vi "CRYAPI MANAGER LIB.vi"(4 "sOption":string, 8 "tFrame":T2, 9 "sData":string, 10 "nData":i32, 11 "sAction":string) -> (1 "nData_Out":i32, 2 "sData_Out":string, 3 "tFrame_Out":T2)   [LabVIEW 2013]
uses:
  <vilib>/Utility/miscctls.llb/LVRectTypeDef.ctl
  CRYMain Sub Window Global.vi
  CRYStepSetup/CRYStepSetup Global.vi
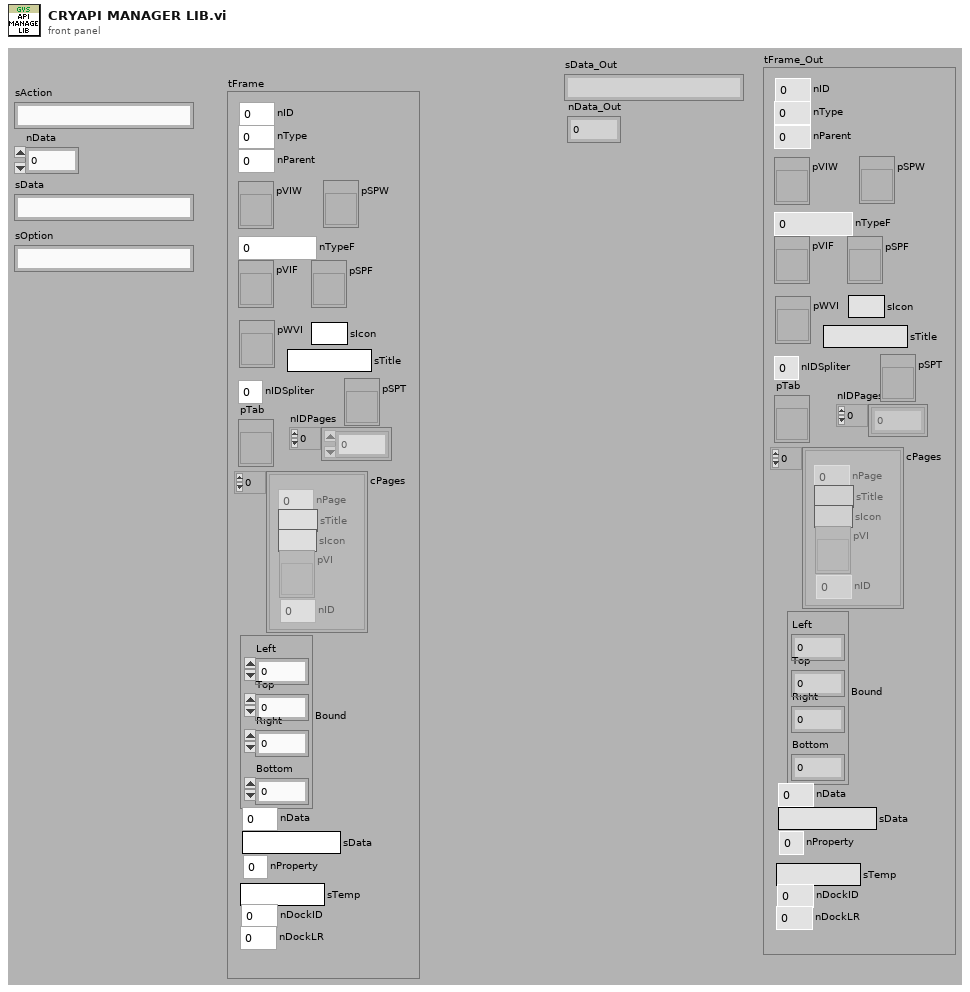
[diagram p1: front panel]
types:
  T1 = typedef "LVRectTypeDef.ctl" = cluster{"Left":i16, "Top":i16, "Right":i16, "Bottom":i16}
  T2 = cluster{"nType":i32, "nParent":i32, "pVIW":refnum<vi>, "pSPW":refnum<vi>, "nTypeF":i32, "pVIF":refnum<vi>, "pSPF":refnum<vi>, "nIDSpliter":i32, "nProperty":i32, "Bound":T1, "nID":i32, "nData":i32, "sData":string, "pWVI":refnum<vi>, "sTitle":string, "cPages":cluster{"nPage":i32, "sTitle":string, "sIcon":string, "pVI":refnum<vi>, "nID":i32}[], "pTab":refnum<vi>, "nIDPages":i32[], "pSPT":refnum<vi>, "sTemp":string, "nDockID":i32, "nDockLR":i32, "sIcon":string}
  T3 = cluster{"nID":i32[], "Frame":cluster{"nType":i32, "nParent":i32, "pVIW":refnum<vi>, "pSPW":refnum<vi>, "nTypeF":i32, "pVIF":refnum<vi>, "pSPF":refnum<vi>, "nIDSpliter":i32, "nProperty":i32, "Bound":T1, "nID":i32, "nData":i32, "sData":string, "pWVI":refnum<vi>, "sTitle":string, "cPages":cluster{"nPage":i32, "sTitle":string, "sIcon":string, "pVI":refnum<vi>, "nID":i32}[], "pTab":refnum<vi>, "nIDPages":i32[], "pSPT":refnum<vi>, "sTemp":string, "nDockID":i32, "nDockLR":i32, "sIcon":string}[]}
  T4 = cluster{"nPos":i32, "Rect":T1, "Sizing":enum16{"Sticks Top/Left", "Sticks Bottom/Right", "Proportional"}}[]
  T5 = cluster{"nPos":i32, "Rect":T1, "Sizing":enum16{"Sticks Top/Left", "Sticks Bottom/Right", "Proportional"}}
  T6 = enum16{"Sticks Top/Left", "Sticks Bottom/Right", "Proportional"}
  T7 = enum32{"Invalid", "Standard", "Closed", "Hidden", "Minimized", "Maximized"}
  T8 = cluster{"nID":i32[], "Spliter":cluster{"nType":i32, "nTypeP":i32, "pVI":refnum<vi>, "pSpliter":refnum<vi>, "pSPL":refnum<vi>, "pVIL":refnum<vi>, "pSPR":refnum<vi>, "pVIR":refnum<vi>, "nIDTL":i32, "nIDL":i32, "nIDTR":i32, "nIDR":i32, "nID":i32, "nIDParent":i32, "nData":i32, "sData":string}[]}
  T9 = cluster{"nType":i32, "nTypeP":i32, "pVI":refnum<vi>, "pSpliter":refnum<vi>, "pSPL":refnum<vi>, "pVIL":refnum<vi>, "pSPR":refnum<vi>, "pVIR":refnum<vi>, "nIDTL":i32, "nIDL":i32, "nIDTR":i32, "nIDR":i32, "nID":i32, "nIDParent":i32, "nData":i32, "sData":string}[]
  T10 = cluster{"nType":i32, "nParent":i32, "pVIW":refnum<vi>, "pSPW":refnum<vi>, "nTypeF":i32, "pVIF":refnum<vi>, "pSPF":refnum<vi>, "nIDSpliter":i32, "nProperty":i32, "Bound":T1, "nID":i32, "nData":i32, "sData":string, "pWVI":refnum<vi>, "sTitle":string, "cPages":cluster{"nPage":i32, "sTitle":string, "sIcon":string, "pVI":refnum<vi>, "nID":i32}[], "pTab":refnum<vi>, "nIDPages":i32[], "pSPT":refnum<vi>, "sTemp":string, "nDockID":i32, "nDockLR":i32, "sIcon":string}[]
  T11 = typedef "CRYWindows Sysem.ctl" = cluster{"cFrame":cluster{"nID":i32[], "Frame":cluster{"nType":i32, "nParent":i32, "pVIW":refnum<vi>, "pSPW":refnum<vi>, "nTypeF":i32, "pVIF":refnum<vi>, "pSPF":refnum<vi>, "nIDSpliter":i32, "nProperty":i32, "Bound":T1, "nID":i32, "nData":i32, "sData":string, "pWVI":refnum<vi>, "sTitle":string, "cPages":cluster{"nPage":i32, "sTitle":string, "sIcon":string, "pVI":refnum<vi>, "nID":i32}[], "pTab":refnum<vi>, "nIDPages":i32[], "pSPT":refnum<vi>, "sTemp":string, "nDockID":i32, "nDockLR":i32, "sIcon":string}[]}, "cSpliter":cluster{"nID":i32[], "Spliter":cluster{"nType":i32, "nTypeP":i32, "pVI":refnum<vi>, "pSpliter":refnum<vi>, "pSPL":refnum<vi>, "pVIL":refnum<vi>, "pSPR":refnum<vi>, "pVIR":refnum<vi>, "nIDTL":i32, "nIDL":i32, "nIDTR":i32, "nIDR":i32, "nID":i32, "nIDParent":i32, "nData":i32, "sData":string}[]}, "ActiveWID":i32, "cSpliterPos":cluster{"nPos":i32, "Rect":T1, "Sizing":enum16{"Sticks Top/Left", "Sticks Bottom/Right", "Proportional"}}[], "CounterWID":i32, "CounterActive":i32, "CounterSpliter":i32, "cWinStatus":cluster{"nData":i32, "nActiveNum":i32}[], "StepName":string, "StepVINo":i32}
  T12 = cluster{"sStepName":string, "nStepVINo":i32, "nStepVINoDisplay":i32}
  T13 = cluster{"nType":i32, "nTypeP":i32, "pVI":refnum<vi>, "pSpliter":refnum<vi>, "pSPL":refnum<vi>, "pVIL":refnum<vi>, "pSPR":refnum<vi>, "pVIR":refnum<vi>, "nIDTL":i32, "nIDL":i32, "nIDTR":i32, "nIDR":i32, "nID":i32, "nIDParent":i32, "nData":i32, "sData":string}
  T14 = cluster{"CLOSE_HIDE":i32, "CLOSE_CLOSE":i32, "DOCK_ENABLE":i32, "DOCK_DISABLE":i32, "FOCUS_SHOW":i32, "FOCUS_HIDE":i32}
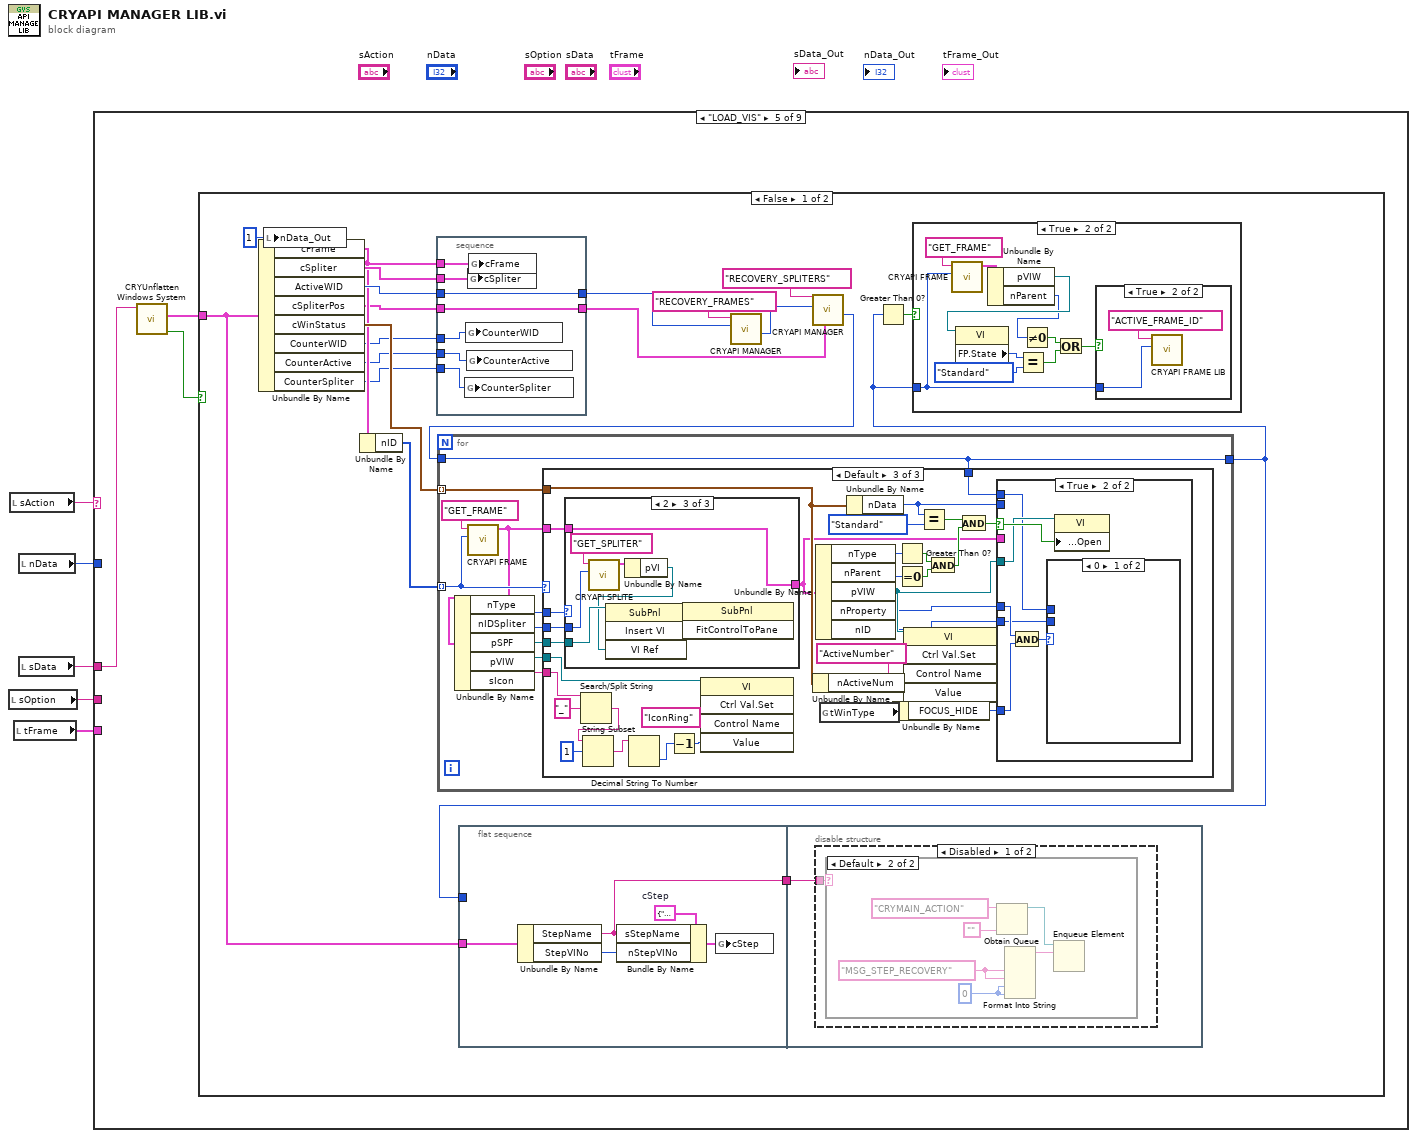
[diagram p0: block diagram]
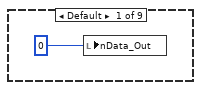
[diagram p2: hidden frame]
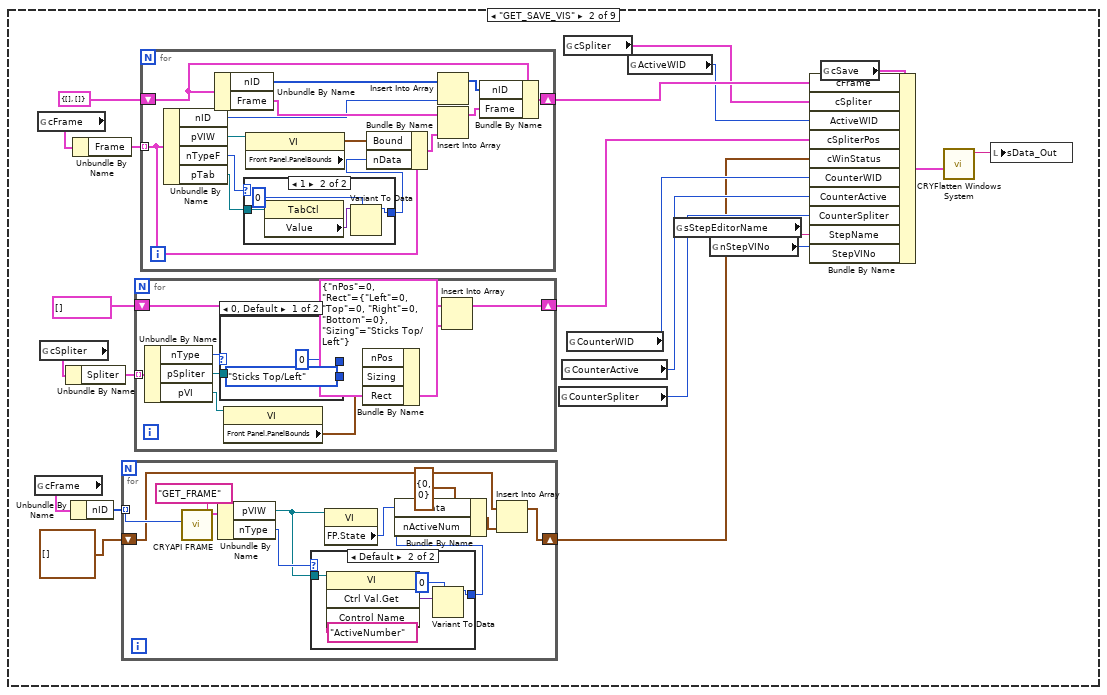
[diagram p3: hidden frame]
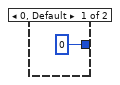
[diagram p4: hidden frame]
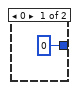
[diagram p5: hidden frame]
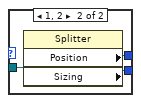
[diagram p6: hidden frame]
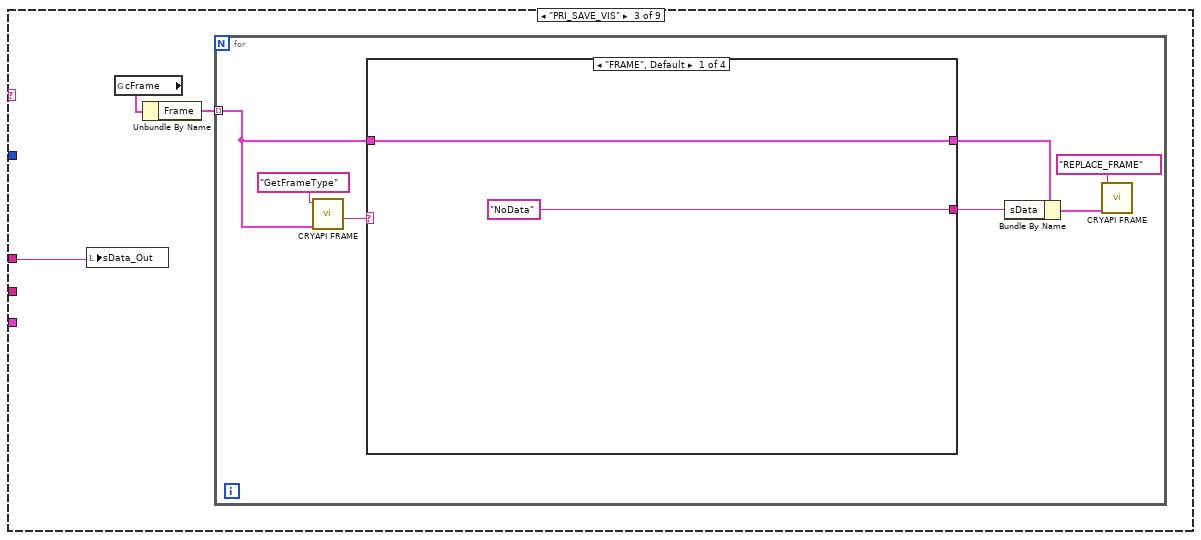
[diagram p7: hidden frame]
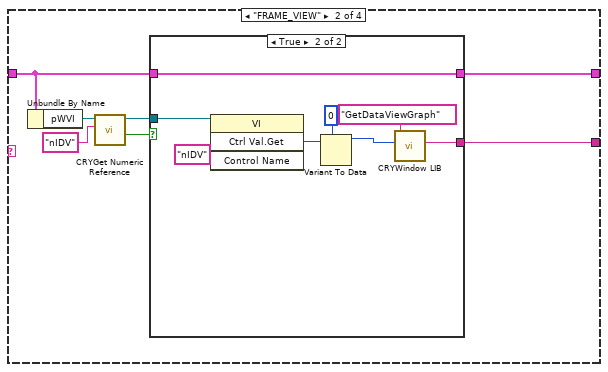
[diagram p8: hidden frame]
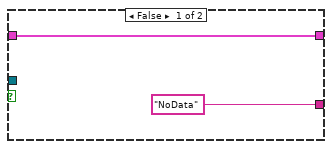
[diagram p9: hidden frame]
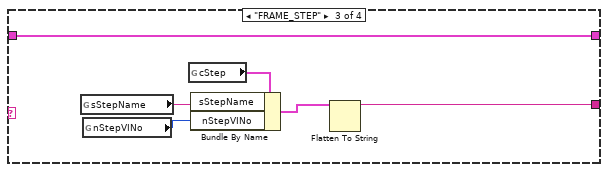
[diagram p10: hidden frame]
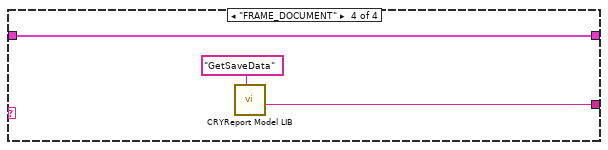
[diagram p11: hidden frame]
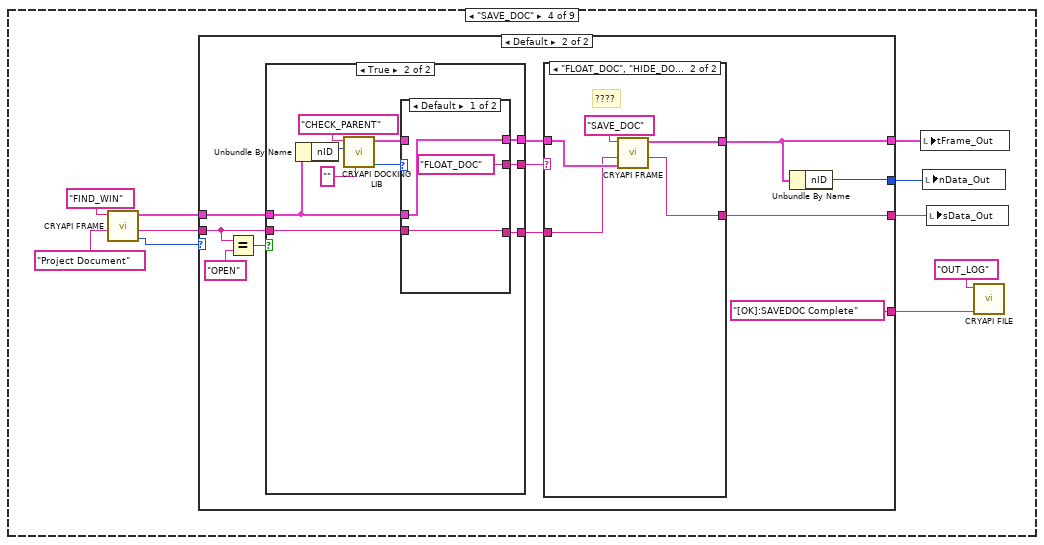
[diagram p12: hidden frame]
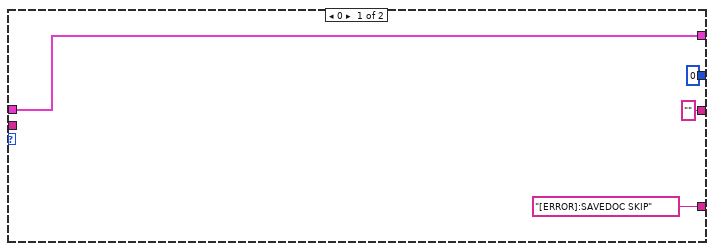
[diagram p13: hidden frame]
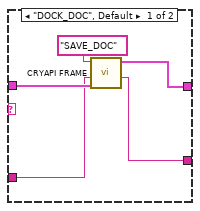
[diagram p14: hidden frame]
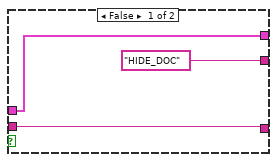
[diagram p15: hidden frame]
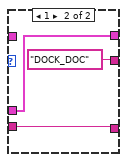
[diagram p16: hidden frame]
diagram:
  n1 = local read "sOption"() -> (w1:string)
  n2 = local read "sAction"() -> (w5:string)
  n3 = local read "tFrame"() -> (w3:T2)
  n4 = local read "nData"() -> (w4:i32)
  n5 = local read "sData"() -> (w2:string)
  n6 = case shown="\"LOAD_VIS\"" w5 {
    selector: w5 -> [_ _ _ _ _ w324 _ _ _]
    tunnel: w4 -> [_ _ _ _ _ _ _ _ _]
    tunnel: w2 -> [_ _ w81 _ w175 w323 _ _ w350]
    tunnel: w3 -> [_ _ _ _ _ w322 _ _ _]
    tunnel: w1 -> [_ _ _ _ _ _ _ _ w348]
    frame Default {
      n7 = local write "nData_Out"(0 ("nData_Out")) -> ()
    }
    frame "GET_SAVE_VIS" {
      n8 = global read "CRYMain Sub Window Global.vi" "cFrame"() -> (w18:T3)
      n9 = global read "CRYMain Sub Window Global.vi" "cFrame"() -> (w22:T3)
      n10 = global read "CRYMain Sub Window Global.vi" "cSpliter"() -> (w14:T8)
      n11 = Unbundle By Name(w14) -> ("Spliter"=w15:T9)
      n12 = Unbundle By Name(w18) -> ("nID"=w17:i32[])
      n13 = Unbundle By Name(w22) -> ("Frame"=w21:T10)
      n14 = for {
        shift-right: [w54] -> w19
        shift-left: cluster{"nData":i32, "nActiveNum":i32}[] [] ("cWinStatus") -> [w55]
        tunnel: w17 -> [w57] mode=indexing
        n15 = call "CRYAPI FRAME.vi"("nData"=w57, "sAction"="GET_FRAME") -> ("tFrame_Out"=w56:T2)  [unwired: 4 in, 5 out]
        n16 = Unbundle By Name(w56) -> ("pVIW"=w48:refnum<vi>, "nType"=w51:i32)
        n17 = case shown="Default" w51 {
          tunnel: [0 ("Numeric") w61] -> w50
          tunnel: w48 -> [_ w60]
          frame 0 {
          }
          frame Default {
            n18 = invoke class="VI" method="Ctrl Val.Get"(reference=w60, "Control Name"="ActiveNumber") -> ("Get Control Value Variant"=w62:variant)  [unwired: 2 in, 3 out]
            n19 = Variant To Data(type=0 ("Numeric"), Variant=w62) -> (data=w61:i32)  [unwired: 1 in, 1 out]
          }
        }
        n20 = property class="VI"(reference=w48) -> ("FP.State"=w49:T7)  [unwired: 1 in, 2 out]
        n21 = Bundle By Name(cluster=cluster{"nData":i32, "nActiveNum":i32} {"nData"=0, "nActiveNum"=0} ("tWinStatus"), "nData"=w49, "nActiveNum"=w50) -> (w52:cluster{"nData":i32, "nActiveNum":i32})
        n22 = Insert Into Array(array=w55, new element=w52) -> (w54:cluster{"nData":i32, "nActiveNum":i32}[])  [unwired: 1 in]
      }
      n23 = for {
        shift-right: [w73] -> w16
        shift-left: T4 [] ("nSpliterPos") -> [w74]
        tunnel: w15 -> [w71] mode=indexing
        n24 = Unbundle By Name(w71) -> ("nType"=w75:i32, "pSpliter"=w72:refnum<vi>, "pVI"=w70:refnum<vi>)
        n25 = case shown="0, Default" w75 {
          tunnel: w72 -> [_ w80]
          tunnel: [0 ("Position") w79] -> w69
          tunnel: [T6."Sticks Top/Left" ("Sizing") w78] -> w65
          frame 0, Default {
          }
          frame 1, 2 {
            n26 = property class="Splitter"(reference=w80) -> ("Position"=w79:i32, "Sizing"=w78:T6)  [unwired: 1 in, 2 out]
          }
        }
        n27 = property class="VI"(reference=w70) -> ("Front Panel.PanelBounds"=w68:T1)  [unwired: 1 in, 2 out]
        n28 = Bundle By Name(cluster=T5 {"nPos"=0, "Rect"={"Left"=0, "Top"=0, "Right"=0, "Bottom"=0}, "Sizing"=enum."Sticks Top/Left"} ("tSpliterSave"), "nPos"=w69, "Sizing"=w65, "Rect"=w68) -> (w67:T5)
        n29 = Insert Into Array(array=w74, new element=w67) -> (w73:T4)  [unwired: 1 in]
      }
      n30 = for {
        tunnel: w21 -> [w41] mode=indexing
        shift-right: [w32] -> w23
        shift-left: T3 {"nID"=[], "Frame"=[]} ("cFrame") -> [w35]
        n31 = Unbundle By Name(w41) -> ("nID"=w36:i32, "pVIW"=w42:refnum<vi>, "nTypeF"=w31:i32, "pTab"=w30:refnum<vi>)
        n32 = Unbundle By Name(w35) -> ("nID"=w39:i32[], "Frame"=w38:T10)
        n33 = case shown="1" w31 {
          tunnel: [0 w46] -> w29
          tunnel: w30 -> [_ w45]
          frame 0, Default {
          }
          frame 1 {
            n34 = property class="TabCtl"(reference=w45) -> ("Value"=w44:variant)  [unwired: 1 in, 2 out]
            n35 = Variant To Data(type=0, Variant=w44) -> (data=w46:i32)  [unwired: 1 in, 1 out]
          }
        }
        n36 = property class="VI"(reference=w42) -> ("Front Panel.PanelBounds"=w40:T1)  [unwired: 1 in, 2 out]
        n37 = Bundle By Name(cluster=w41, "Bound"=w40, "nData"=w29) -> (w37:T2)
        n38 = Insert Into Array(array=w39, new element=w36) -> (w34:i32[])  [unwired: 1 in]
        n39 = Insert Into Array(array=w38, new element=w37) -> (w33:T10)  [unwired: 1 in]
        n40 = Bundle By Name(cluster=w35, "nID"=w34, "Frame"=w33) -> (w32:T3)
      }
      n41 = global read "CRYMain Sub Window Global.vi" "CounterSpliter"() -> (w26:i32)
      n42 = global read "CRYMain Sub Window Global.vi" "CounterActive"() -> (w25:i32)
      n43 = global read "CRYMain Sub Window Global.vi" "cSpliter"() -> (w12:T8)
      n44 = global read "CRYMain Sub Window Global.vi" "CounterWID"() -> (w24:i32)
      n45 = global read "CRYMain Sub Window Global.vi" "ActiveWID"() -> (w13:i32)
      n46 = global read "CRYStepSetup Global.vi" "sStepEditorName"() -> (w8:string)
      n47 = global read "CRYStepSetup Global.vi" "nStepVINo"() -> (w7:i32)
      n48 = global read "CRYMain Sub Window Global.vi" "cSave"() -> (w11:T11)
      n49 = Bundle By Name(cluster=w11, "cFrame"=w23, "cSpliter"=w12, "ActiveWID"=w13, "cSpliterPos"=w16, "cWinStatus"=w19, "CounterWID"=w24, "CounterActive"=w25, "CounterSpliter"=w26, "StepName"=w8, "StepVINo"=w7) -> (w10:T11)
      n50 = call "CRYFlatten Windows System.vi"("Windows System"=w10) -> ("WinSys flattened"=w9:string)  [unwired: 10 in]
      n51 = local write "sData_Out"(w9) -> ()
    }
    frame "PRI_SAVE_VIS" {
      n52 = local write "sData_Out"(w81) -> ()
      n53 = global read "CRYMain Sub Window Global.vi" "cFrame"() -> (w83:T3)
      n54 = Unbundle By Name(w83) -> ("Frame"=w82:T10)
      n55 = for {
        tunnel: w82 -> [w89] mode=indexing
        n56 = call "CRYAPI FRAME.vi"("tFrame"=w89, "sAction"="GetFrameType") -> ("sData_Out"=w88:string)  [unwired: 6 in, 3 out]
        n57 = case shown="\"FRAME\", Default" w88 {
          tunnel: w89 -> [w92 w95 w115 w118]
          tunnel: [w92 w94 w115 w118] -> w84
          tunnel: ["NoData" ("sData_Out") w93 w110 w116] -> w87
          frame "FRAME", Default {
          }
          frame "FRAME_VIEW" {
            n58 = Unbundle By Name(w95) -> ("pWVI"=w98:refnum<vi>)
            n59 = call "CRYGet Numeric Reference.vi"("Label Name"="nIDV", "VI Refnum"=w98) -> ("Boolean"=w97:bool, "VI Refnum Out"=w96:refnum<vi>)  [unwired: 7 in, 1 out]
            n60 = case shown="True" w97 {
              tunnel: w96 -> [_ w107]
              tunnel: w95 -> [w101 w104]
              tunnel: ["NoData" ("sData_Out") w105] -> w93
              tunnel: [w101 w104] -> w94
              frame False {
              }
              frame True {
                n61 = invoke class="VI" method="Ctrl Val.Get"(reference=w107, "Control Name"="nIDV") -> ("Get Control Value Variant"=w109:variant)  [unwired: 2 in, 3 out]
                n62 = Variant To Data(type=0, Variant=w109) -> (data=w102:i32)  [unwired: 1 in, 1 out]
                n63 = call "CRYWindow LIB.vi"("nData"=w102, "sAction"="GetDataViewGraph") -> ("sData_Out"=w105:string)  [unwired: 9 in]
              }
            }
          }
          frame "FRAME_STEP" {
            n64 = global read "CRYStepSetup Global.vi" "sStepName"() -> (w113:string)
            n65 = global read "CRYStepSetup Global.vi" "nStepVINo"() -> (w112:i32)
            n66 = global read "CRYStepSetup Global.vi" "cStep"() -> (w114:T12)
            n67 = Bundle By Name(cluster=w114, "sStepName"=w113, "nStepVINo"=w112) -> (w111:T12)
            n68 = Flatten To String(anything=w111) -> (data string=w110:string)  [unwired: 1 in, 4 out]
          }
          frame "FRAME_DOCUMENT" {
            n69 = call "CRYReport Model LIB.vi"("sAction"="GetSaveData") -> ("sData_Out"=w116:string)  [unwired: 9 in, 1 out]
          }
        }
        n70 = Bundle By Name(cluster=w84, "sData"=w87) -> (w85:T2)
        n71 = call "CRYAPI FRAME.vi"("tFrame"=w85, "sAction"="REPLACE_FRAME") -> ()  [unwired: 6 in, 4 out]
      }
    }
    frame "SAVE_DOC" {
      n72 = call "CRYAPI FRAME.vi"("sData"="Project Document" ("Window Type"), "sAction"="FIND_WIN") -> ("nData_Out"=w122:i32, "sData_Out"=w123:string, "tFrame_Out"=w126:T2)  [unwired: 4 in, 3 out]
      n73 = case shown="Default" w122 {
        tunnel: w126 -> [w132 w143]
        tunnel: [w132 w137] -> w125
        tunnel: [0 w142] -> w124
        tunnel: w123 -> [_ w135]
        tunnel: ["" ("sData_Out") w136] -> w121
        tunnel: ["[ERROR]:SAVEDOC SKIP" ("sData") "[OK]:SAVEDOC Complete" ("sData")] -> w119
        frame 0 {
        }
        frame Default {
          n74 = Equal?(x=w135, y="OPEN") -> (x = y?=w141:bool)
          n75 = case shown="True" w141 {
            tunnel: w143 -> [w156 w162]
            tunnel: [w156 w160] -> w138
            tunnel: ["HIDE_DOC" w159] -> w139
            tunnel: w135 -> [w154 w158]
            tunnel: [w154 w157] -> w134
            frame False {
            }
            frame True {
              n76 = Unbundle By Name(w162) -> ("nID"=w161:i32)
              n77 = call "CRYAPI DOCKING LIB.vi"("sData"="", "nData"=w161, "sAction"="CHECK_PARENT") -> ("nData_Out"=w164:i32, "tFrame_Out"=w163:T2)  [unwired: 2 in, 5 out]
              n78 = case shown="Default" w164 {
                tunnel: w162 -> [w168 w172]
                tunnel: w163 -> [_ _]
                tunnel: [w168 w172] -> w160
                tunnel: ["FLOAT_DOC" "DOCK_DOC"] -> w159
                tunnel: [w167 w170] -> w157
                tunnel: w158 -> [w167 w170]
                frame Default {
                }
                frame 1 {
                }
              }
            }
          }
          n79 = case shown="\"FLOAT_DOC\", \"HIDE_DOC\"" w139 {
            tunnel: w138 -> [w147 w152]
            tunnel: [w146 w150] -> w137
            tunnel: [w145 w149] -> w136
            tunnel: w134 -> [w144 w151]
            frame "DOCK_DOC", Default {
              n80 = call "CRYAPI FRAME.vi"("tFrame"=w147, "sData"=w144, "sAction"="SAVE_DOC") -> ("sData_Out"=w145:string, "tFrame_Out"=w146:T2)  [unwired: 3 in, 4 out]
            }
            frame "FLOAT_DOC", "HIDE_DOC" {
              # "????"
              n81 = call "CRYAPI FRAME.vi"("tFrame"=w152, "sData"=w151, "sAction"="SAVE_DOC") -> ("sData_Out"=w149:string, "tFrame_Out"=w150:T2)  [unwired: 3 in, 4 out]
            }
          }
          n82 = Unbundle By Name(w137) -> ("nID"=w142:i32)
        }
      }
      n83 = local write "tFrame_Out"(w125) -> ()
      n84 = local write "nData_Out"(w124) -> ()
      n85 = local write "sData_Out"(w121) -> ()
      n86 = call "CRYAPI FILE.vi"("sData"=w119, "sAction"="OUT_LOG") -> ()  [unwired: 8 in, 2 out]
    }
    frame "LOAD_VIS" {
      n87 = call "CRYUnflatten Windows System.vi"("Flatten WinSys"=w175) -> ("Error?"=w174:bool, "Windows System"=w173:T11)  [unwired: 8 in, 1 out]
      n88 = case shown="False" w174 {
        tunnel: w173 -> [w176 _]
        frame False {
          n89 = Unbundle By Name(w176) -> ("cFrame"=w186:T3, "cSpliter"=w187:T8, "ActiveWID"=w195:i32, "cSpliterPos"=w185:T4, "cWinStatus"=w189:cluster{"nData":i32, "nActiveNum":i32}[], "CounterWID"=w183:i32, "CounterActive"=w182:i32, "CounterSpliter"=w181:i32)
          n90 = local write "nData_Out"(1 ("nData_Out")) -> ()
          n91 = Unbundle By Name(w186) -> ("nID"=w190:i32[])
          n92 = stacked-sequence {
            tunnel: w195 -> [w213]
            tunnel: w187 -> [w215]
            tunnel: w186 -> [w214]
            tunnel: [w213] -> w188
            tunnel: [w212] -> w184
            tunnel: w185 -> [w212]
            tunnel: w183 -> [w211]
            tunnel: w182 -> [w210]
            tunnel: w181 -> [w209]
            frame #0 {
              n93 = global write "CRYMain Sub Window Global.vi" "CounterSpliter"(w209) -> ()
              n94 = global write "CRYMain Sub Window Global.vi" "CounterWID"(w211) -> ()
              n95 = global write "CRYMain Sub Window Global.vi" "CounterActive"(w210) -> ()
              n96 = global write "CRYMain Sub Window Global.vi" "cSpliter"(w215) -> ()
              n97 = global write "CRYMain Sub Window Global.vi" "cFrame"(w214) -> ()
            }
          }
          n98 = flat-sequence {
            tunnel: w178 -> [_]
            tunnel: [w198] -> w177
            tunnel: w176 -> [w196]
            tunnel: w177 -> [w201]
            frame #0 {
              w200 = T12 {"sStepName"="", "nStepVINo"=0, "nStepVINoDisplay"=0}  # cStep
              n99 = Unbundle By Name(w196) -> ("StepName"=w198:string, "StepVINo"=w197:i32)
              n100 = Bundle By Name(cluster=w200, "sStepName"=w198, "nStepVINo"=w197) -> (w199:T12)
              n101 = global write "CRYStepSetup Global.vi" "cStep"(w199) -> ()
            }
            frame #1 {
              n102 = disable-structure shown="Disabled" {
                disable-tunnel: w201 -> [w202 _]
                frame Disabled {
                  n103 = case shown="Default" w202 {
                    frame "NoData" {
                    }
                    frame Default {
                      w203 = 0 ("input 3")
                      w208 = "MSG_STEP_RECOVERY" ("input 1")
                      n104 = Obtain Queue(name (unnamed)="CRYMAIN_ACTION" ("YAxisTitle"), element data type="" ("Action Type")) -> (queue out=w207:refnum<queue>)  [unwired: 3 in, 2 out]
                      n105 = Format Into String(w208, w208, w203, w203) -> (resulting string=w206:string)  [unwired: 3 in, 1 out]
                      n106 = Enqueue Element(queue=w207, element=w206) -> ()  [unwired: 1 in, 4 out]
                    }
                  }
                }
                frame Enabled {
                }
              }
            }
          }
          n107 = call "CRYAPI MANAGER.vi"("nData"=w188, "sAction"="RECOVERY_FRAMES") -> ("nData_Out"=w191:i32)  [unwired: 3 in, 6 out]
          n108 = call "CRYAPI MANAGER.vi"("cSpliterPos"=w184, "nData"=w191, "sAction"="RECOVERY_SPLITERS") -> ("nData_Out"=w179:i32)  [unwired: 2 in, 6 out]
          n109 = for {
            tunnel: w190 -> [w235] mode=indexing
            tunnel: w189 -> [w237] mode=indexing
            tunnel: [w228] -> w178
            tunnel: w179 -> [w228]
            n110 = call "CRYAPI FRAME.vi"("nData"=w235, "sAction"="GET_FRAME") -> ("tFrame_Out"=w234:T2)  [unwired: 4 in, 5 out]
            n111 = Unbundle By Name(w234) -> ("nType"=w233:i32, "nIDSpliter"=w232:i32, "pSPF"=w231:refnum<vi>, "pVIW"=w230:refnum<vi>, "sIcon"=w229:string)
            n112 = case shown="Default" w235 {
              tunnel: w237 -> [_ _ w273]
              tunnel: w234 -> [w245 w252 w277]
              tunnel: w233 -> [_ _ w280]
              tunnel: w232 -> [_ _ w279]
              tunnel: w231 -> [_ _ w278]
              tunnel: w230 -> [_ _ w265]
              tunnel: w229 -> [_ _ w264]
              tunnel: w228 -> [_ _ w257]
              frame 1 {
                n113 = Unbundle By Name(w245) -> ("nID"=w248:i32, "pVIW"=w251:refnum<vi>, "pVIF"=w250:refnum<vi>, "pSPF"=w244:refnum<vi>, "nIDSpliter"=w242:i32)
                n114 = global write "CRYMain Sub Window Global.vi" "MainFrame_nID"(w248) -> ()
                n115 = global write "CRYMain Sub Window Global.vi" "MainFrame_VIRef"(w251) -> ()
                n116 = global write "CRYMain Sub Window Global.vi" "MsgProVI"(w250) -> ()
                n117 = call "CRYAPI SPLITE.vi"("nData"=w242, "sAction"="GET_SPLITER") -> ("tSpliter_Out"=w241:T13)  [unwired: 4 in, 5 out]
                n118 = Unbundle By Name(w241) -> ("pVI"=w240:refnum<vi>)
                n119 = global read "CRYMain Sub Window Global.vi" "Main View SubPanel"() -> (w247:refnum<vi>)
                n120 = invoke class="SubPnl" method="Insert VI"(reference=w244, "VI Ref"=w240) -> (reference out=w239:refnum<vi>, error out=w238:errorcluster)  [unwired: 2 in, 2 out]
                n121 = invoke class="SubPnl" method="Insert VI"(reference=w247, "VI Ref"=w251) -> (reference out=w246:refnum<vi>, error out=w249:errorcluster)  [unwired: 2 in, 2 out]
                n122 = invoke class="SubPnl" method="FitControlToPane"(reference=w239, error in=w238) -> ()  [unwired: 1 in, 3 out]
                n123 = invoke class="SubPnl" method="FitControlToPane"(reference=w246, error in=w249) -> ()  [unwired: 1 in, 3 out]
              }
              frame 2 {
                n124 = Unbundle By Name(w252) -> ("pVIW"=w253:refnum<vi>, "nID"=w254:i32)
                n125 = global write "CRYMain Sub Window Global.vi" "MainTabVI"(w253) -> ()
                n126 = global write "CRYMain Sub Window Global.vi" "MainTabID"(w254) -> ()
              }
              frame Default {
                n127 = case shown="2" w280 {
                  tunnel: w279 -> [_ _ w299]
                  tunnel: w278 -> [_ _ w298]
                  tunnel: [w287 w290 w294] -> w256
                  tunnel: w277 -> [w287 w290 w294]
                  frame 0, Default {
                  }
                  frame 1 {
                    n128 = Unbundle By Name(w290) -> ("nTypeF"=w292:i32, "pTab"=w289:refnum<vi>)
                    n129 = Equal?(x=w292, y=1) -> (x = y?=w288:bool)
                    n130 = case shown="True" w288 {
                      tunnel: w289 -> [_ w293]
                      frame False {
                      }
                      frame True {
                        n131 = invoke class="TabCtl" method="FitControlToPane"(reference=w293) -> ()  [unwired: 2 in, 3 out]
                      }
                    }
                  }
                  frame 2 {
                    n132 = call "CRYAPI SPLITE.vi"("nData"=w299, "sAction"="GET_SPLITER") -> ("tSpliter_Out"=w300:T13)  [unwired: 4 in, 5 out]
                    n133 = Unbundle By Name(w300) -> ("pVI"=w297:refnum<vi>)
                    n134 = invoke class="SubPnl" method="Insert VI"(reference=w298, "VI Ref"=w297) -> (reference out=w296:refnum<vi>, error out=w295:errorcluster)  [unwired: 2 in, 2 out]
                    n135 = invoke class="SubPnl" method="FitControlToPane"(reference=w296, error in=w295) -> ()  [unwired: 1 in, 3 out]
                  }
                }
                n136 = Search/Split String(string=w264, search string/char (-)="_" ("search string")) -> (match + rest of string=w269:string)  [unwired: 3 out]
                n137 = String Subset(string=w269, offset (0)=1) -> (substring=w267:string)  [unwired: 1 out]
                n138 = Decimal String To Number(string=w267) -> (number=w263:i32)  [unwired: 3 out]
                n139 = Decrement(x=w263) -> (x-1=w266:i32)
                n140 = invoke class="VI" method="Ctrl Val.Set"(reference=w265, "Control Name"="IconRing", "Value"=w266) -> ()  [unwired: 2 in, 5 out]
                n141 = Unbundle By Name(w273) -> ("nActiveNum"=w274:i32)
                n142 = Unbundle By Name(w256) -> ("nType"=w286:i32, "nParent"=w283:i32, "pVIW"=w272:refnum<vi>, "nProperty"=w260:i32, "nID"=w258:i32)
                n143 = global read "CRYMain Sub Window Global.vi" "tWinType"() -> (w262:T14)
                n144 = Unbundle By Name(w273) -> ("nData"=w255:i32)
                n145 = Unbundle By Name(w262) -> ("FOCUS_HIDE"=w259:i32)
                n146 = Greater Than 0?(x=w286) -> (x > 0?=w282:bool)
                n147 = Equal To 0?(x=w283) -> (x = 0?=w261:bool)
                n148 = invoke class="VI" method="Ctrl Val.Set"(reference=w272, "Control Name"="ActiveNumber", "Value"=w274) -> ()  [unwired: 2 in, 5 out]
                n149 = Equal?(x=w255, y=T7."Standard" ("Front Panel Window:State")) -> (x = y?=w284:bool)
                n150 = And(x=w282, y=w261) -> (x .and. y?=w281:bool)
                n151 = And(x=w284, y=w281) -> (x .and. y?=w285:bool)
                n152 = case shown="True" w285 {
                  selector: w285 -> [_ w313]
                  tunnel: w272 -> [_ w312]
                  tunnel: w260 -> [_ w311]
                  tunnel: w259 -> [_ w310]
                  tunnel: w258 -> [_ w309]
                  tunnel: w257 -> [_ w307]
                  tunnel: w256 -> [w302 _]
                  tunnel: w255 -> [w304 _]
                  frame False {
                    n153 = Equal?(x=w304, y=T7."Closed" ("Front Panel Window:State")) -> (x = y?=w303:bool)
                    n154 = case shown="True" w303 {
                      tunnel: w302 -> [_ w306]
                      frame False {
                      }
                      frame True {
                        n155 = call "CRYPIC SHOW FRAME.vi"("tFrame"=w306) -> ()  [unwired: 10 in, 1 out]
                      }
                    }
                  }
                  frame True {
                    n156 = And(x=w311, y=w310) -> (x .and. y?=w308:i32)
                    n157 = case shown="0" w308 {
                      tunnel: w309 -> [_ w318]
                      tunnel: w307 -> [_ w320]
                      frame 0 {
                      }
                      frame Default {
                        n158 = Equal?(x=w320, y=w318) -> (x = y?=w317:bool)
                        n159 = Select(t="ACTIVE_FALSE" ("sAction"), s=w317, f="INACTIVE_TRUE" ("sAction")) -> (s? t:f=w314:string)
                        n160 = call "CRYAPI FRAME LIB.vi"("sData"=w314, "nData"=w318, "sAction"="SET_PINSTATE") -> ()  [unwired: 3 in, 6 out]
                      }
                    }
                    n161 = property class="VI"(reference=w312, "Front Panel.Open"=w313) -> ()  [unwired: 1 in, 2 out]
                  }
                }
              }
            }
          }
          n162 = Greater Than 0?(x=w178) -> (x > 0?=w180:bool)
          n163 = case shown="True" w180 {
            tunnel: w178 -> [_ w220]
            frame False {
            }
            frame True {
              n164 = call "CRYAPI FRAME.vi"("nData"=w220, "sAction"="GET_FRAME") -> ("tFrame_Out"=w224:T2)  [unwired: 4 in, 5 out]
              n165 = Unbundle By Name(w224) -> ("pVIW"=w223:refnum<vi>, "nParent"=w219:i32)
              n166 = property class="VI"(reference=w223) -> ("FP.State"=w221:T7)  [unwired: 1 in, 2 out]
              n167 = Equal?(x=w221, y=T7."Standard" ("Front Panel Window:State")) -> (x = y?=w216:bool)
              n168 = Not Equal To 0?(x=w219) -> (x != 0?=w217:bool)
              n169 = Or(x=w217, y=w216) -> (x .or. y?=w218:bool)
              n170 = case shown="True" w218 {
                tunnel: w220 -> [_ w226]
                frame False {
                }
                frame True {
                  n171 = call "CRYAPI FRAME LIB.vi"("nData"=w226, "sAction"="ACTIVE_FRAME_ID") -> ()  [unwired: 4 in, 6 out]
                }
              }
            }
          }
        }
        frame True {
          n172 = local write "nData_Out"(0 ("nData_Out")) -> ()
        }
      }
    }
    frame "ACTIVE_FRAME" {
      n173 = call "CRYAPI FRAME LIB.vi"("tFrame"=w322, "sData"=w323, "sAction"=w324) -> ()  [unwired: 3 in, 6 out]
      n174 = local write "tFrame_Out"(w322) -> ()
    }
    frame "CLOSE_ALL_FRAME" {
      n175 = while {
        stop <- w328 stop-if-true
        n176 = global read "CRYMain Sub Window Global.vi" "cFrame"() -> (w329:T3)
        n177 = Unbundle By Name(w329) -> ("nID"=w327:i32[])
        n178 = Array Size(array=w327) -> (size(s)=w326:i32)
        n179 = Equal To 0?(x=w326) -> (x = 0?=w328:bool)
        n180 = case shown="False" w328 {
          tunnel: w327 -> [w337 _]
          tunnel: w326 -> [w335 _]
          frame False {
            n181 = Decrement(x=w335) -> (x-1=w334:i32)
            n182 = Index Array(array=w337, index=w334) -> (element=w333:i32)
            n183 = call "CRYPIC GET FRAME.vi"("nID"=w333) -> ("tFrame_Out"=w332:T2)  [unwired: 8 in, 2 out]
            n184 = call "CRYPIC Save StepView.vi"("sAction"="SetNoSaveStepView", "tFrame"=w332) -> ("tFrame_Out"=w330:T2)  [unwired: 9 in]
            n185 = call "CRYPART CLOSE FRAME.vi"("sAction"="CloseFrameBytFrame", "tFrame"=w330) -> ()  [unwired: 10 in]
          }
          frame True {
          }
        }
        n186 = Wait (ms)(milliseconds to wait=u32 10) -> ()  [unwired: 1 out]
      }
    }
    frame "DETACH_ALL_TAB" {
      n187 = global read "CRYMain Sub Window Global.vi" "cFrame"() -> (w339:T3)
      n188 = Unbundle By Name(w339) -> ("Frame"=w338:T10)
      n189 = for {
        tunnel: w338 -> [w340] mode=indexing
        n190 = Unbundle By Name(w340) -> ("nTypeF"=w341:i32)
        n191 = case shown="1" w341 {
          tunnel: w340 -> [_ w342]
          frame Default {
          }
          frame 1 {
            n192 = Unbundle By Name(w342) -> ("pSPW"=w344:refnum<vi>, "pSPF"=w343:refnum<vi>)
            n193 = invoke class="SubPnl" method="Remove VI"(reference=w343) -> ()  [unwired: 2 in, 3 out]
            n194 = invoke class="SubPnl" method="Remove VI"(reference=w344) -> ()  [unwired: 2 in, 3 out]
          }
        }
      }
    }
    frame "FIND_WINDOW" {
      n195 = call "CRYPIC PreGetVIName.vi"("sVIName"=w348) -> ("sData_Out"=w345:string, "sVIName_Out"=w346:string)  [unwired: 9 in]
      n196 = case shown="Default" w346 {
        tunnel: w350 -> [w355 w359]
        tunnel: [w355 w358] -> w349
        tunnel: w348 -> [_ w360]
        tunnel: ["FIND_WIN_STEMP" ("sAction") w357] -> w347
        tunnel: w345 -> [_ w356]
        frame Default {
        }
        frame "StepView" {
          n197 = case shown="\"\"" w356 {
            tunnel: w360 -> [w362 _]
            tunnel: w359 -> [_ w364]
            tunnel: [w362 w364] -> w358
            tunnel: ["FIND_WIN_STEMP" ("sAction") "FIND_WIN_TITLE" ("sAction")] -> w357
            frame Default {
            }
            frame "" {
            }
          }
        }
      }
      n198 = call "CRYAPI FRAME.vi"("sData"=w349, "sAction"=w347) -> ("nData_Out"=w352:i32, "sData_Out"=w351:string, "tFrame_Out"=w353:T2)  [unwired: 4 in, 3 out]
      n199 = local write "sData_Out"(w351) -> ()
      n200 = local write "tFrame_Out"(w353) -> ()
      n201 = local write "nData_Out"(w352) -> ()
    }
  }
